vi "Dashboard Main.vi"() -> ()   [LabVIEW 2020]
uses:
  <vilib>/event_ctls.llb/eventvkey.ctl
  <vilib>/Rock Robotics/Network Tables/NT Read Numeric Array.vi
  <vilib>/Rock Robotics/WPI/Dashboard/WPI_DashboardLogging Global.vi
panel:
  out "Camera Perf":string
  in  "Camera Settings":T1={"Frame Rate"=30, "Compression"=30, "Size"=1, "DB Camera Config"=FALSE} {"Frame Rate" scale=1.0..30.0; "Compression" scale=100.0..-1.0; "Size" items=["640x480", "320x240", "160x120"]}
  in  "TCP":refnum<k5>
  in  "Rec Mode":enum32{"Stop", "Record", "Playback"}(radio)
  out "Robot IP":string
  out "Image Message":string="Timeout in Camera Communications"
  in  "Dashboard Tab":T2(tab)
  in  "Select Auto":string(combo)="Select Autonomous ..."
  out "NT Connection":bool
  out "MotorChart R":cluster{"Numeric":dbl, "Numeric":dbl}(graph)
  out "MotorChart L":cluster{"Numeric":dbl, "Numeric":dbl}(graph)
  out "MotorSliders R":cluster{"MotorSlide1":dbl, "MotorSlide2":dbl} {"MotorSlide2" scale=-1.0..1.0 scale format="%#_2e"; "MotorSlide1" scale=-1.0..1.0 scale format="%#_2e"}
  out "MotorSliders L":cluster{"MotorSlide1":dbl, "MotorSlide2":dbl} {"MotorSlide2" scale=-1.0..1.0 scale format="%#_2e"; "MotorSlide1" scale=-1.0..1.0 scale format="%#_2e"}
  out "Gyro":dbl(knob) scale=0.0..360.0
  out "JS1 Z":dbl(slide) scale=-1.0..1.0 scale format="%#_2e"
  out "JS1 Graph":cluster{"X":dbl, "Y":dbl}[](graph)
  out "JS1 Buttons":T3
  out "JS2 Z":dbl(slide) scale=-1.0..1.0 scale format="%#_2e"
  out "JS2 Graph":cluster{"X":dbl, "Y":dbl}[](graph)
  out "JS2 Buttons":T3
  out "Mode":T4(ring)=enum."Auto Disabled"
  out "Right Camera Perf":cluster{"Bandwidth (Mbps)":dbl, "FPS":dbl}
  in  "DB/String 9":string
  in  "DB/String 8":string
  in  "DB/String 7":string
  in  "DB/String 6":string
  in  "DB/String 5":string
  in  "DB/String 4":string
  in  "DB/String 3":string
  in  "DB/String 2":string
  in  "DB/String 1":string
  in  "DB/String 0":string
  in  "DB/Slider 0":dbl(slide) scale=0.0..5.0
  in  "DB/Slider 1":dbl(slide) scale=0.0..5.0
  in  "DB/Slider 2":dbl(slide) scale=0.0..5.0
  in  "DB/Slider 3":dbl(slide) scale=0.0..5.0
  out "DB/LED 3":bool
  out "DB/LED 2":bool
  out "DB/LED 1":bool
  out "DB/LED 0":bool
  in  "DB/Button 3":bool
  in  "DB/Button 2":bool
  in  "DB/Button 1":bool
  in  "DB/Button 0":bool caption="New Name"
  in  "Test Slider":dbl(slide) scale=0.0..100.0 scale format="%#_3g"
  in  "On/Off":bool caption="Solenoid"
  in  "Test Name":u16(ring) items=["Select the test to run..."]
  in  "Test Tree":string(tree)
  in  "Motor":cluster{"Value":dbl, "Enable":bool} {"Value" scale=-1.0..1.0 scale format="%#_3g"}
  out "Progress":T5 {"Test Progress" scale=0.0..100.0}
  in  "Rev/Fwd":cluster{"Forward":bool, "Reverse":bool}
  in  "Test Ring":u16(ring) items=["Monochrome", "Color"]
  in  "CheckList":i32(listbox)
  out "Tree":string(tree)
  out "Camera Image":T6(plugin-control)
  out "Background":bool
  in  "Camera Name":string(combo)="No Camera Selection"
  # "HW"
  # "Joysticks"
  # "Drive Motors"
  # "Front"
  # "Right"
  # "Left"
  # "Back"
  # "This tab is a great place for autonomous settings and robot-specific values.\nPlace controls and indicators inside this tab and match name to\nDashboard Variables on robot. You can also delete this comment."
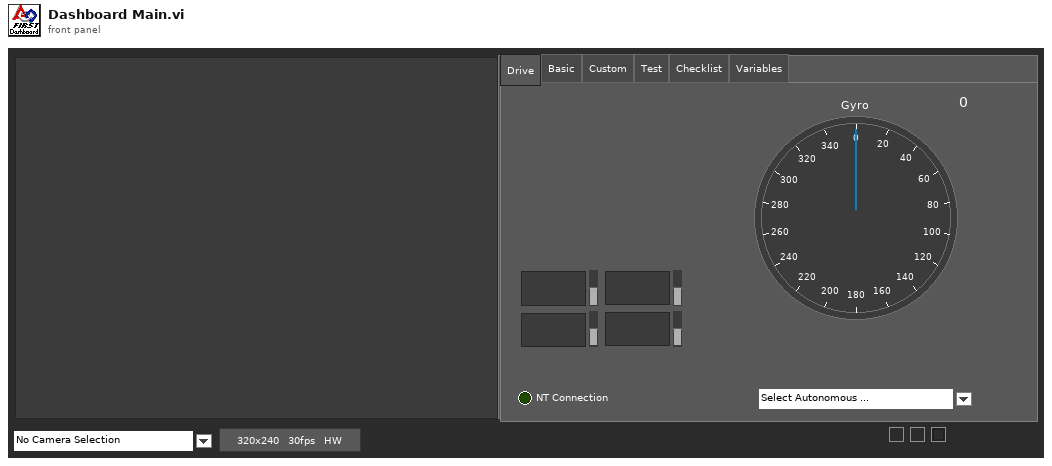
[diagram p1: front panel]
types:
  T1 = cluster{"Frame Rate":i32, "Compression":i32, "Size":u16, "DB Camera Config":bool}
  T2 = enum32{"Drive", "Basic", "Custom", "Test", "Checklist", "Variables"}
  T3 = cluster{bool, bool, bool, bool, bool, bool, bool, bool, bool, bool, bool, bool}
  T4 = enum8{"Tele-Op Disabled", "Tele-Op Enabled", "Auto Disabled", "Auto Enabled", "Test Disabled", "Test Enabled", "Disconnected", "No Code", "E-Stop"}
  T5 = cluster{"Test Progress":u8, "Test Progress Text":string}
  T6 = typedef "IMAQ Image.ctl" = refnum<image>
  T7 = cluster{"Save Path":path, "Interval (s)":dbl, "Keep":i32}
  T8 = enum32{"Drive", "Camera", "Basic", "Custom", "Test", "Commands", "Checklist", "Variables"}
  T9 = typedef "Image Type" = u32
  T10 = cluster{"Error Strings":string, "Disable Counts":cluster{u16, u16}, "Rail Faults":cluster{u16, u16, u16}, "Robot IP":string, "DB Mode":u8, "Event Info":cluster{"Name":string, "Type":u8, "Number":u16, "Replay":u8}}
  T11 = cluster{"Storage":cluster{"Disk Free":u64, "RAM Block":u32, "RAM free":u32}, "CPU Utilization":cluster{"CPU % ISR":sgl, "CPU % Time Crit":sgl, "CPU % Timed Str":sgl, "CPU % High":sgl, "CPU % Above":sgl, "CPU % Normal":sgl, "CPU % Low":sgl}, "CAN":cluster{"% Bus Utilization":sgl, "Bus Off Cnt":u32, "TX_FIFO Full Cnt":u32, "Receive Error Cnt":u8, "Transmit Error Cnt":u8}, "HID":cluster{"HID Outputs":u32, "Rumble Low":u16, "Rumble High":u16}[]}
  T12 = cluster{"Status bits":cluster{"Test Mode":bool, "Autonomous":bool, "Enabled":bool, "Code Start":bool, "Brownout":bool, "Reserved 2":bool, "Reserved 3":bool, "E-Stop":bool}, "Code Trace":cluster{"Disabled":bool, "TeleOp":bool, "Auto":bool, "Test":bool}, "Controller Type":enum16{"unknown", "cRIO", "roboRio"}, "Code?":enum16{"unknown", "noCode", "code"}, "Battery V":dbl}
  T13 = cluster{"Control Bits":cluster{"TestMode":bool, "Autonomous":bool, "Enabled":bool, "FMS Present":bool, bool, bool, bool, "E-Stop":bool}, "Team Station ":u8, "Countdown":sgl, "Joystick Values":cluster{"Axes":dbl[], "Buttons":bool[], "POVs":i16[]}[]}
  T14 = cluster{"Axes":dbl[], "Buttons":bool[], "POVs":i16[]}[]
  T15 = cluster{"Axes":dbl[], "Buttons":bool[], "POVs":i16[]}
  T16 = cluster{"Buttons[0]":bool, "Buttons[1]":bool, "Buttons[2]":bool, "Buttons[3]":bool, "Buttons[4]":bool, "Buttons[5]":bool, "Buttons[6]":bool, "Buttons[7]":bool, "Buttons[8]":bool, "Buttons[9]":bool, "Buttons[10]":bool, "Buttons[11]":bool}
  T17 = cluster{"Camera Image":refnum<vi>, "Dashboard Tab":refnum<vi>, "Background":refnum<vi>, "Rec Mode":refnum<vi>, "Test Slider":refnum<vi>, "On/Off ":refnum<vi>, "Test Ring":refnum<vi>, "Rev/Fwd":refnum<vi>, "Test Name":refnum<vi>, "Motor":refnum<vi>, "Progress":refnum<vi>, "CheckList":refnum<vi>, "Tree":refnum<vi>, "Test Tree":refnum<vi>, "Camera Settings":refnum<vi>, "Camera Name":refnum<vi>, "Camera Perf":refnum<vi>, "Camera Settings":refnum<vi>, "Camera Name":refnum<vi>, "Camera Image":refnum<vi>}
  T18 = cluster{"Global Rectangle":i32[], "Contours":cluster{"Contour Type":u32, "ROI Type":u32, "Points":i32[]}[]}
  T19 = cluster{"Camera Name":string, string, "Saved DB Images Info":cluster{"Save Path":path, "Interval (s)":dbl, "Keep":i32}}
  T20 = cluster{"Operation":enum16{"Update", "Clear"}, "Color Box":u32}[]
  T21 = typedef "eventvkey.ctl" = enum16{"ASCII", "Enter", "Return", "Shift", "Ctrl", "Alt", "Cmd", "Opt", "Caps", "NumLock", "Clear", "Break", "Up", "Down", "Left", "Right", "Insert", "Delete", "Home", "End", "PageUp", "PageDown", "Escape", "Help", "Pause", "ScrollLock", "F1", "F2", "F3", "F4", "F5", "F6", "F7", "F8", "F9", "F10", "F11", "F12", "F13", "F14", "F15", "F16", "F17", "F18", "F19", "F20", "F21", "F22", "F23", "F24", "Play", "VolumeUp", "VolumeDown", "Mute", "Two Byte Char"}
  T22 = cluster{"Image Size":bool, "Image Type":bool, "Pixel Value":bool, "ROI Information":bool, "Zoom Factor":bool}
  T23 = cluster{"Operation":enum16{"Update", "Clear"}, "Color Box":u32}
  T24 = cluster{"Shift":bool, "Ctrl":bool, "Alt":bool, "Cmd":bool, "Opt":bool}
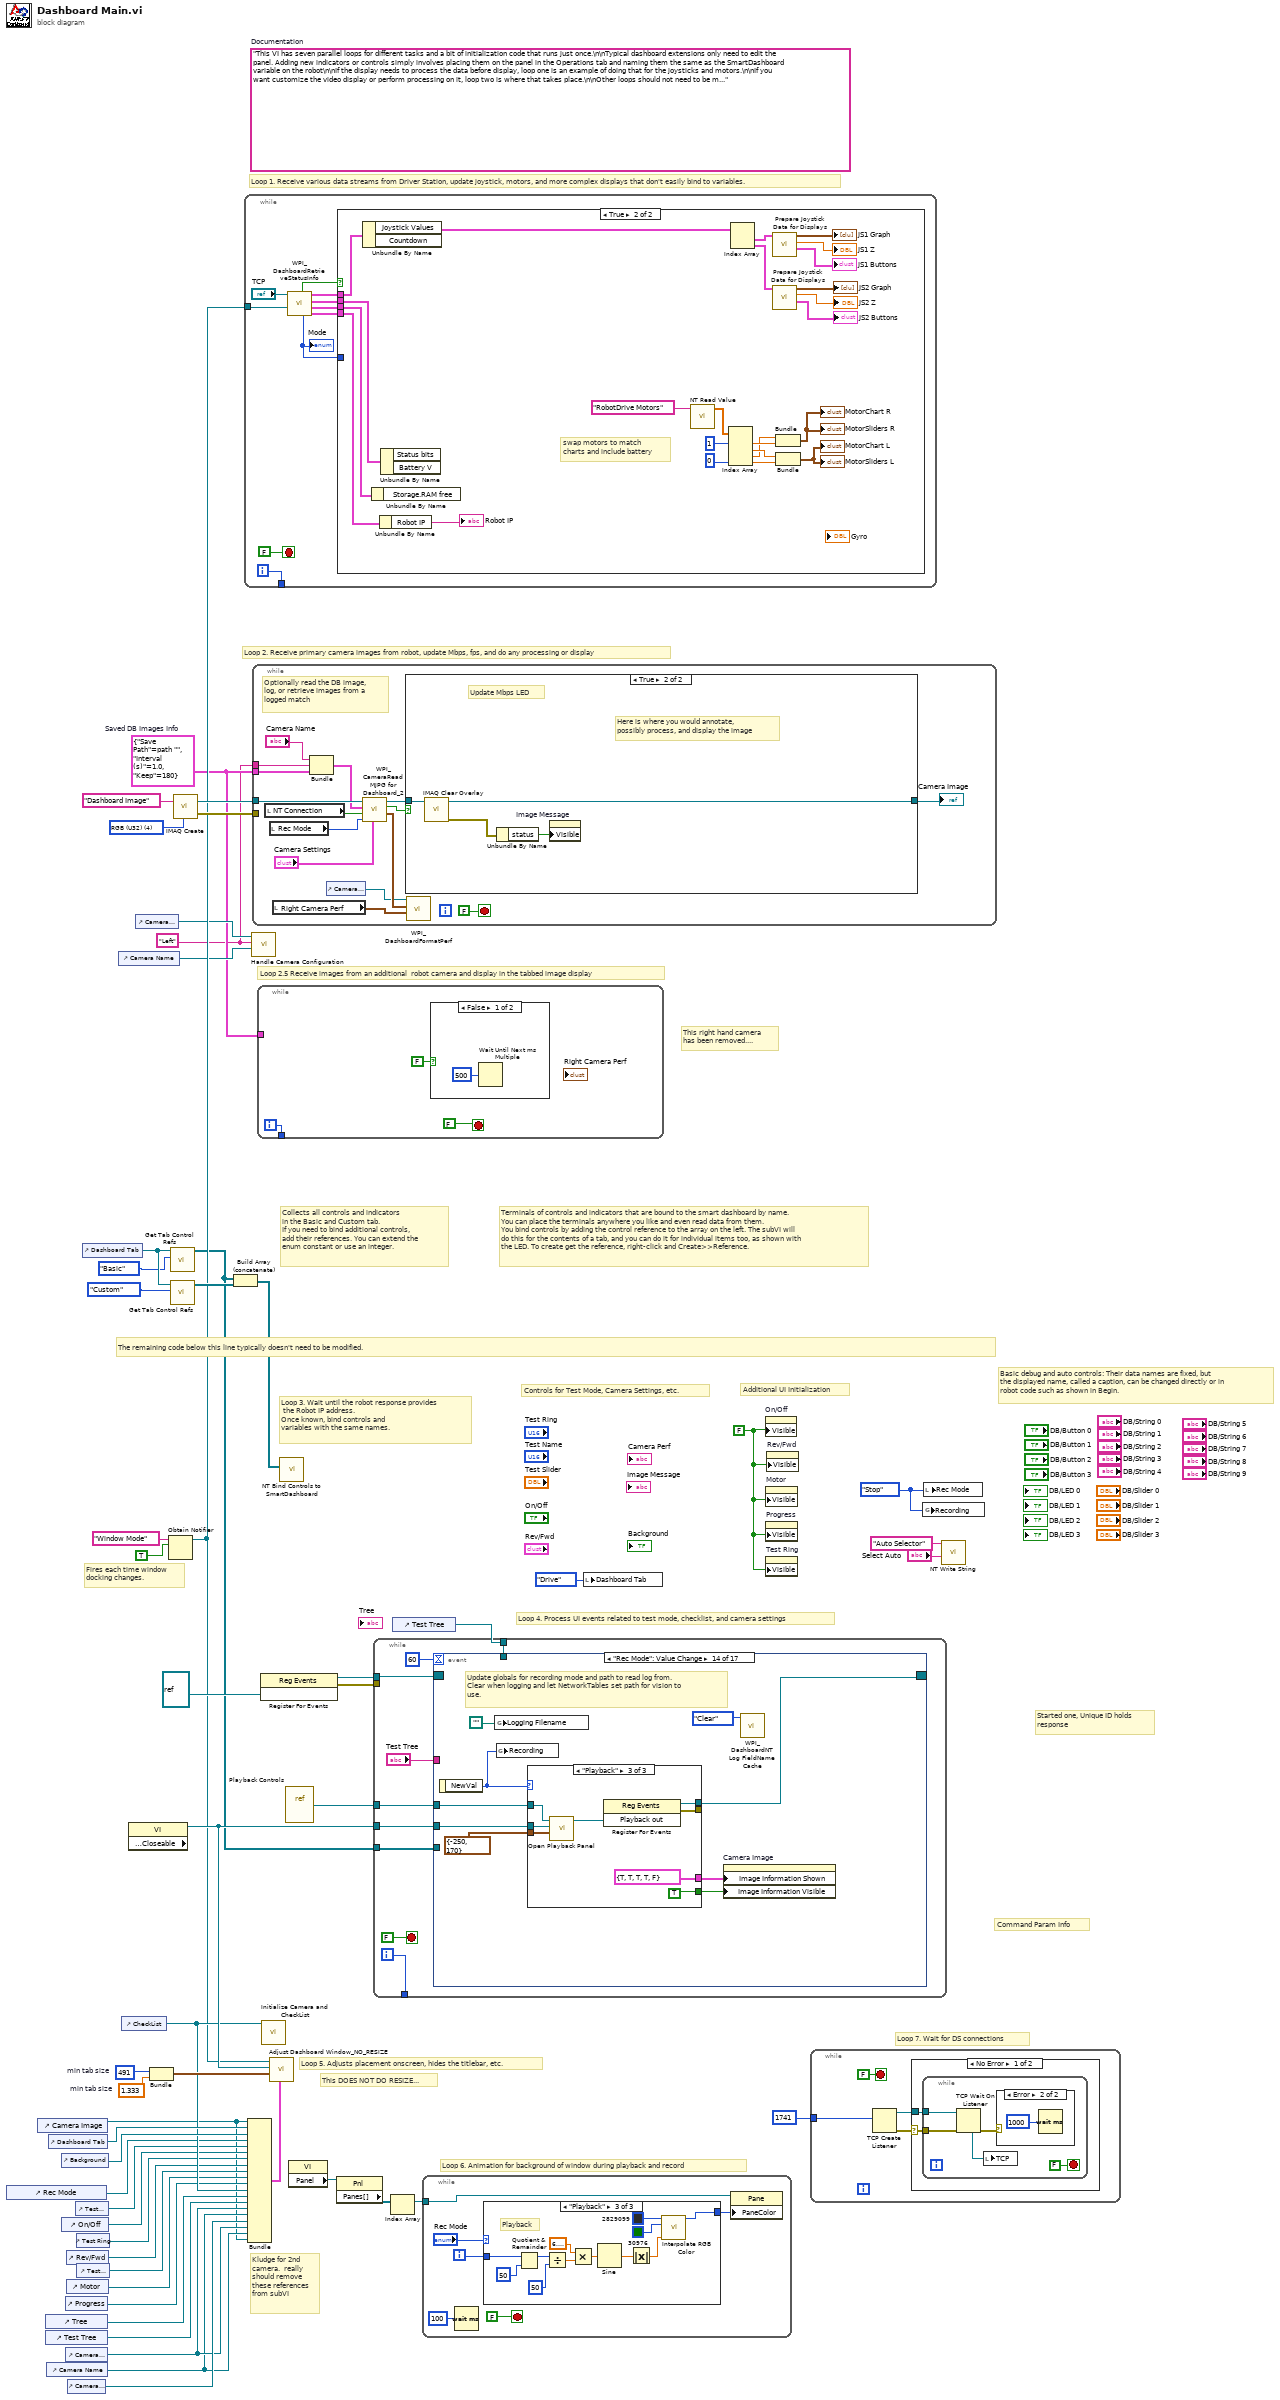
[diagram p0: block diagram]
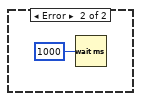
[diagram p4: hidden frame]
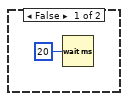
[diagram p5: hidden frame]
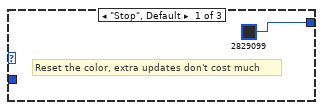
[diagram p6: hidden frame]
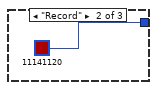
[diagram p7: hidden frame]
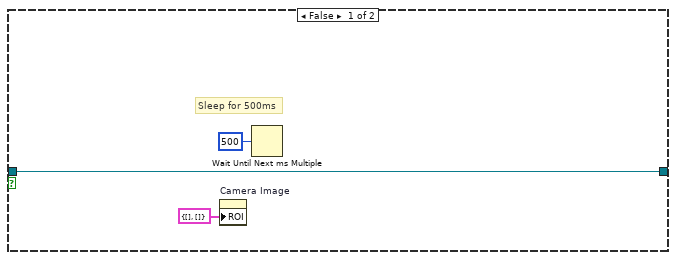
[diagram p8: hidden frame]
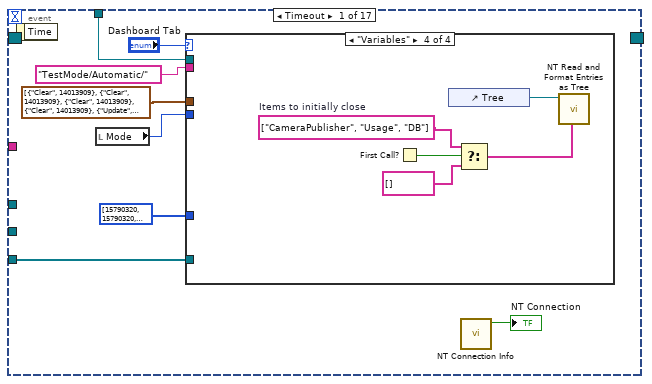
[diagram p9: hidden frame]
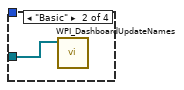
[diagram p11: hidden frame]
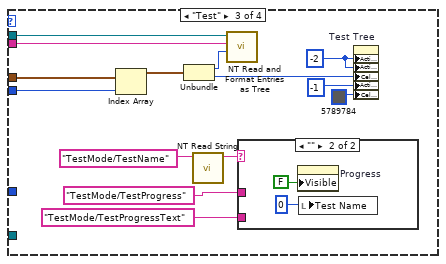
[diagram p12: hidden frame]
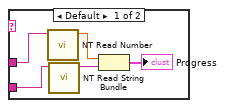
[diagram p13: hidden frame]
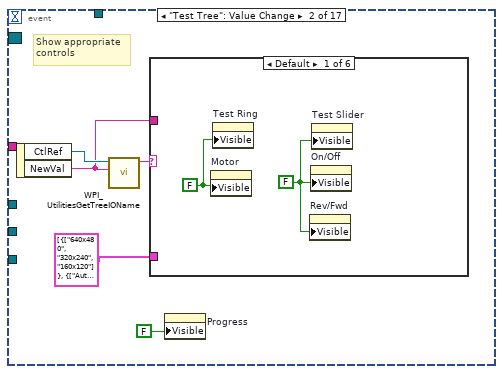
[diagram p14: hidden frame]
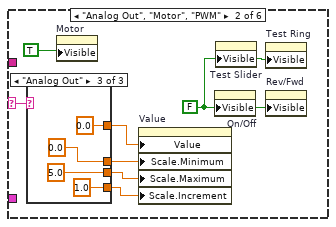
[diagram p15: hidden frame]
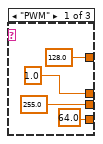
[diagram p16: hidden frame]
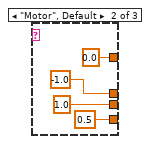
[diagram p17: hidden frame]
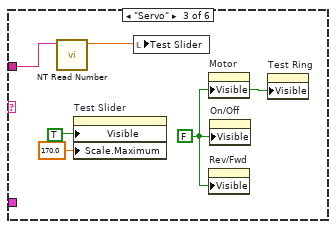
[diagram p18: hidden frame]
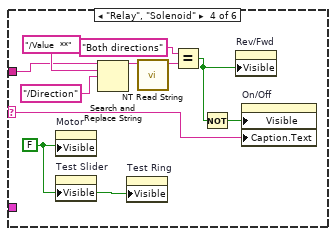
[diagram p19: hidden frame]
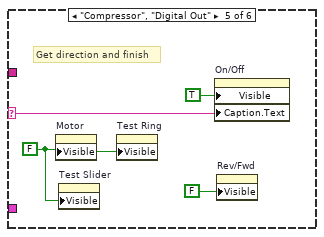
[diagram p20: hidden frame]
diagram:
  w6 = T7 {"Save Path"=path "", "Interval (s)"=1.0, "Keep"=180}  # Saved DB Images Info
  w5 = "Left"
  w33 = 491  # min tab size
  w32 = 1.333  # min tab size
  w39 = enum32{"Stop", "Record", "Playback"}."Stop" ("Rec Mode")
  w17 = FALSE ("Visible")
  (unwired) "This VI has seven parallel loops for different tasks and a bit of initialization code that runs just once.\n\nTypical dashboard extensions only need to edit the panel. Adding new indicators or controls simply involves placing them on the panel in the Operations tab and naming them the same as the SmartDashboard variable on the robot\n\nIf the display needs to process the data before display, loop one is an example of doing that for the joysticks and motors.\n\nIf you want customize the video display or perform processing on it, loop two is where that takes place.\n\nOther loops should not need to be modified. They are pretty standard, and document the task they perform."  # Documentation
  w53 = T9 4 items=["Grayscale (U8)", "Grayscale (I16)", "Grayscale (SGL)", "Complex (CSG)", "RGB (U32)", "HSL (U32)", "RGB (U64)"] ("Image Type")
  # "Kludge for 2nd\ncamera.  really\nshould remove\nthese references\nfrom subVI"
  # "This right hand camera\nhas been removed...."
  # "This DOES NOT DO RESIZE..."
  # "Loop 2.5 Receive images from an additional  robot camera and display in the tabbed image display"
  # "Command Param Info"
  # "Started one, Unique ID holds\nresponse"
  # "Loop 7. Wait for DS connections"
  # "Basic debug and auto controls: Their data names are fixed, but\nthe displayed name, called a caption, can be changed directly or in\nrobot code such as shown in Begin."
  # "Controls for Test Mode, Camera Settings, etc."
  # "Additional UI Initialization"
  # "Loop 6. Animation for background of window during playback and record"
  # "Fires each time window\ndocking changes."
  # "Collects all controls and indicators\nin the Basic and Custom tab.\nIf you need to bind additional controls,\nadd their references. You can extend the\nenum constant or use an integer."
  # "The remaining code below this line typically doesn't need to be modified."
  # "Loop 4. Process UI events related to test mode, checklist, and camera settings"
  # "Terminals of controls and indicators that are bound to the smart dashboard by name.\nYou can place the terminals anywhere you like and even read data from them.\nYou bind controls by adding the control reference to the array on the left. The subVI will\ndo this for the contents of a tab, and you can do it for individual items too, as shown with\nthe LED. To create get the reference, right-click and Create>>Reference."
  # "Loop 3. Wait until the robot response provides\n the Robot IP address.\nOnce known, bind controls and\nvariables with the same names."
  # "Loop 5. Adjusts placement onscreen, hides the titlebar, etc."
  # "Loop 1. Receive various data streams from Driver Station, update joystick, motors, and more complex displays that don't easily bind to variables."
  # "Loop 2. Receive primary camera images from robot, update Mbps, fps, and do any processing or display"
  n1 = control-ref of="Rec Mode"() -> (w23:refnum<vi>)
  n2 = control-ref of="Camera Image"() -> (w2:refnum<vi>)
  n3 = control-ref of="Tree"() -> (w27:refnum<vi>)
  n4 = control-ref of="Test Tree"() -> (w26:refnum<vi>)
  n5 = control-ref of="Camera Name"() -> (w3:refnum<vi>)
  n6 = control-ref of="Dashboard Tab"() -> (w34:refnum<vi>)
  n7 = control-ref of="Background"() -> (w30:refnum<vi>)
  n8 = control-ref of="On/Off"() -> (w21:refnum<vi>)
  n9 = control-ref of="Progress"() -> (w18:refnum<vi>)
  n10 = control-ref of="Camera Settings"() -> (w4:refnum<vi>)
  n11 = control-ref of="Rev/Fwd"() -> (w19:refnum<vi>)
  n12 = control-ref of="Motor"() -> (w24:refnum<vi>)
  n13 = control-ref of="Camera Perf"() -> (w12:refnum<vi>)
  n14 = control-ref of="Test Slider"() -> (w22:refnum<vi>)
  n15 = control-ref of="Test Ring"() -> (w20:refnum<vi>)
  n16 = control-ref of="Test Name"() -> (w25:refnum<vi>)
  n17 = control-ref of="Dashboard Tab"() -> (w37:refnum<vi>)
  n18 = control-ref of="Camera Name"() -> (w13:refnum<vi>)
  n19 = control-ref of="CheckList"() -> (w28:refnum<vi>)
  n20 = property class="VI" props=["Front Panel.Closeable"]() -> (reference out=w38:refnum<vi>)  [unwired: 2 in, 2 out]
  n21 = control-ref of="Camera Settings"() -> (w14:refnum<vi>)
  n22 = Bundle("min tab size"=w33, "min tab size"=w32) -> (w31:cluster{"min tab size":i32, "min tab size":dbl})  [unwired: 1 in]
  n23 = Obtain Notifier(name (unnamed)="Window Mode", notification data type=TRUE) -> (notifier out=w16:refnum<notifier>)  [unwired: 2 in, 2 out]
  n24 = call <vilib>:"Get Tab Control Refs.vi"("Page Index"=T8."Basic" ("Dashboard Tab"), "TabControl in"=w37) -> ("ControlsOnPage"=w11:refnum<vi>[])  [unwired: 9 in]
  n25 = call <vilib>:"Get Tab Control Refs.vi"("Page Index"=T8."Custom" ("Dashboard Tab"), "TabControl in"=w37) -> ("ControlsOnPage"=w36:refnum<vi>[])  [unwired: 9 in]
  n26 = call "IMAQ Create"("Image Name"="Dashboard Image", "Image Type"=w53) -> ("New Image"=w51:T6, "error out"=w50:errorcluster)  [unwired: 2 in, 1 out]
  n27 = Build Array (concatenate)(w11, w36) -> (w35:refnum<vi>[])
  n28 = while {
    tunnel: [w62] -> _
    tunnel: w16 -> [w54]
    i -> [w62]
    stop <- FALSE stop-if-true
    n29 = call <vilib>:"WPI_DashboardRetrieveStatusInfo.vi"("Window Mode Notifier"=w54, "TCP Cnx"="TCP") -> ("Power and Errors"=w57:T10, "Robot Metrics"=w60:T11, "Status Info"=w61:T12, "Control Info"=w58:T13, "Robot Mode"=w56:T4, "Process?"=w59:bool)  [unwired: 4 in]
    "Mode" <- w56
    n30 = case shown="True" w59 {
      tunnel: w61 -> [_ w88]
      tunnel: w60 -> [_ w87]
      tunnel: w58 -> [_ w86]
      tunnel: w57 -> [_ w85]
      tunnel: w56 -> [_ _]
      frame False {
        n31 = Wait (ms)(milliseconds to wait=u32 20) -> ()  [unwired: 1 out]
      }
      frame True {
        # "swap motors to match\ncharts and include battery"
        n32 = Unbundle By Name(w86) -> ("Joystick Values"=w76:T14)  [unwired: 1 out]
        n33 = Unbundle By Name(w87) -> ()  [unwired: 1 out]
        n34 = Unbundle By Name(w85) -> ("Robot IP"=→"Robot IP":string)
        n35 = Unbundle By Name(w88) -> ()  [unwired: 2 out]
        n36 = call-poly <vilib>:"NT Read Value.vi"("name"="RobotDrive Motors" ("Name")) -> ("value"=w66:dbl[])  [unwired: 8 in, 2 out]
        n37 = Index Array(array=w66, index #1=1, index #4=0) -> (element #1=w80:dbl, element #2=w81:dbl, element #3=w79:dbl, element #4=w84:dbl)  [unwired: 2 in]
        n38 = Index Array(array=w76) -> (element #1=w75:T15, element #2=w71:T15)  [unwired: 2 in]
        n39 = call "Prepare Joystick Data for Displays.vi"("Joystick Values"=w71) -> ("Buttons"=→"JS2 Buttons":T16, "Z Axis"=→"JS2 Z":dbl, "Cartesian Data"=→"JS2 Graph":cluster{"X axis":dbl, "X axis":dbl}[])  [unwired: 8 in]
        n40 = call "Prepare Joystick Data for Displays.vi"("Joystick Values"=w75) -> ("Buttons"=→"JS1 Buttons":T16, "Z Axis"=→"JS1 Z":dbl, "Cartesian Data"=→"JS1 Graph":cluster{"X axis":dbl, "X axis":dbl}[])  [unwired: 8 in]
        n41 = Bundle("Numeric"=w79, "Numeric"=w80) -> (→"MotorChart R" →"MotorSliders R":cluster{"Numeric":dbl, "Numeric":dbl})  [unwired: 1 in]
        n42 = Bundle("Numeric"=w81, "Numeric"=w84) -> (→"MotorChart L" →"MotorSliders L":cluster{"Numeric":dbl, "Numeric":dbl})  [unwired: 1 in]
      }
    }
  }
  n43 = Bundle("Camera Image"=w2, "Dashboard Tab"=w34, "Background"=w30, "Rec Mode"=w23, "Test Slider"=w22, "On/Off"=w21, "Test Ring"=w20, "Rev/Fwd"=w19, "Test Name"=w25, "Motor"=w24, "Progress"=w18, "CheckList"=w28, "Tree"=w27, "Test Tree"=w26, "Camera Settings"=w4, "Camera Name"=w3, "Camera Perf"=w12, "Camera Settings"=w4, "Camera Name"=w3, "Camera Image"=w2) -> (w29:T17)  [unwired: 1 in]
  n44 = call "Handle Camera Configuration.vi"("CameraNameRef"=w13, "Display Name"=w5, "ClusterRef"=w14) -> ()  [unwired: 9 in]
  n45 = while {
    tunnel: w51 -> [w102]
    tunnel: w50 -> [_]
    tunnel: w6 -> [w95]
    tunnel: w5 -> [w92]
    stop <- FALSE stop-if-true
    # "Optionally read the DB image,\nlog, or retrieve images from a\nlogged match"
    n46 = local read "NT Connection"() -> (w96:bool)
    n47 = local read "Rec Mode"() -> (w99:enum32{"Stop", "Record", "Playback"})
    n48 = local read "Right Camera Perf"() -> (w90:cluster{"Bandwidth (Mbps)":dbl, "FPS":dbl})
    n49 = Bundle("Camera Name"="Camera Name", w92, "Saved DB Images Info"=w95) -> (w94:T19)  [unwired: 1 in]
    n50 = control-ref of="Camera Perf"() -> (w89:refnum<vi>)
    n51 = call <vilib>:"WPI_CameraRead MJPG for Dashboard_2.vi"("Camera Settings"="Camera Settings", "Rec Mode"=w99, "NT Connection"=w96, "Capture Info"=w94, "Image in"=w102) -> ("perf info"=w91:cluster{"Bandwidth (Mbps)":dbl, "fps":dbl}, "Active"=w100:bool, "Image\\ out"=w101:T6)  [unwired: 4 in]
    n52 = case shown="True" w100 {
      tunnel: w101 -> [w105 w108]
      tunnel: [w105 w107] -> w97
      frame False {
        # "Sleep for 500ms"
        n53 = property on="Camera Image" class="ImageControl"("ROI"=T18 {"Global Rectangle"=[], "Contours"=[]}) -> ()  [unwired: 2 in, 2 out]
        n54 = Wait Until Next ms Multiple(millisecond multiple=u32 500) -> ()  [unwired: 1 out]
      }
      frame True {
        # "Here is where you would annotate,\npossibly process, and display the image"
        # "Update Mbps LED"
        n55 = call "IMAQ Clear Overlay"("Image"=w108) -> ("error out"=w109:errorcluster, "Image Out"=w107:T6)  [unwired: 2 in, 7 out]
        n56 = Unbundle By Name(w109) -> ("status"=w110:bool)
        n57 = property on="Image Message" class="Str"("Visible"=w110) -> ()  [unwired: 2 in, 2 out]
      }
    }
    "Camera Image" <- w97
    n58 = call <vilib>:"WPI_DashboardFormatPerf.vi"("Right Camera Perf"=w90, "Performance"=w91, "String in"=w89) -> ()  [unwired: 9 in]
  }
  n59 = while {
    tunnel: [w112] -> _
    tunnel: w6 -> [_]
    i -> [w112]
    stop <- FALSE stop-if-true
    n60 = case shown="False" FALSE {
      frame False {
        n61 = Wait Until Next ms Multiple(millisecond multiple=u32 500) -> ()  [unwired: 1 out]
      }
      frame True {
      }
    }
  }
  n62 = register-events(refnum<vi> refnum) -> (reference out=w42:refnum<event-registration>, error out=w41:errorcluster)  [unwired: 2 in]
  n63 = call "Initialize Camera and CheckList.vi"("ListBox in"=w28) -> ()  [unwired: 11 in]
  n64 = call "Adjust Dashboard Window_NO_RESIZE.vi"("Sizing Refnums"=w29, "Size Constraints"=w31, "VI"=w38, "WIn Mode"=w16) -> ()  [unwired: 8 in]
  n65 = call <vilib>:"NT Bind Controls to SmartDashboard.vi"("Bound Control Refs"=w35) -> ()  [unwired: 11 in]
  n66 = vi-ref "Playback Controls.vi"() -> (w43:refnum<vi>)
  n67 = property class="VI"() -> ("Panel"=w45:refnum<vi>)  [unwired: 2 in, 2 out]
  n68 = property class="Pnl"(reference=w45) -> ("Panes[]"=w46:refnum<vi>[])  [unwired: 1 in, 2 out]
  n69 = Index Array(array=w46) -> (element=w44:refnum<vi>)  [unwired: 1 in]
  n70 = control-ref of="Test Tree"() -> (w47:refnum<vi>)
  n71 = while {
    tunnel: [w120] -> _
    tunnel: w47 -> [w119]
    tunnel: w43 -> [w118]
    tunnel: w42 -> [w117]
    tunnel: w41 -> [_]
    tunnel: w38 -> [w116]
    tunnel: w11 -> [w115]
    i -> [w120]
    stop <- FALSE stop-if-true
    n72 = event shown="[13] \"Rec Mode\": Value Change" {
      selector: w117 -> [_ _ _ _ _ _ _ _ _ _ _ _ _ _ _ _ _]
      dyn-events: [_ _ _ _ _ _ _ _ _ _ _ _ _ w325 _ _ _] -> _
      timeout: u32 60 ("milliseconds to wait") -> [_ _ _ _ _ _ _ _ _ _ _ _ _ _ _ _ _]
      tunnel: w119 -> [w130 _ _ _ _ _ _ _ _ _ _ _ _ _ _ _ _]
      tunnel: "Test Tree" -> [_ _ _ _ _ _ _ _ w298 w305 w306 w309 w316 _ _ _ _]
      tunnel: w118 -> [_ _ _ _ _ _ _ _ _ _ _ _ _ w327 _ w342 _]
      tunnel: w116 -> [_ _ _ _ _ _ _ _ _ _ _ _ _ w323 _ _ _]
      tunnel: w115 -> [w125 _ _ _ _ _ _ _ _ _ _ _ _ _ _ _ _]
      event Timeout {
        n73 = event-data() -> ()  [unwired: 1 in, 1 out]
        n74 = local read "Mode"() -> (w128:T4)
        n75 = case shown="\"Variables\"" "Dashboard Tab" {
          tunnel: w130 -> [_ _ w146 _]
          tunnel: "TestMode/Automatic/" ("Name Pattern") -> [_ _ w145 _]
          tunnel: T20 [{"Operation"=enum."Clear", "Color Box"=14013909}, {"Operation"=enum."Clear", "Color Box"=14013909}, {"Operation"=enum."Clear", "Color Box"=14013909}, {"Operation"=enum."Clear", "Color Box"=14013909}, {"Operation"=enum."Update", "Color Box"=14013909}, {"Operation"=enum."Update", "Color Box"=16777215}, {"Operation"=enum."Clear", "Color Box"=14013909}, {"Operation"=enum."Clear", "Color Box"=14013909}, {"Operation"=enum."Clear", "Color Box"=14013909}] -> [_ _ w138 _]
          tunnel: w128 -> [_ _ w137 _]
          tunnel: u32[] [15790320, 15790320, 15790320, 15790320, 16777215, 16777215, 15790320, 15790320, 15790320] -> [_ _ _ _]
          tunnel: w125 -> [_ w132 _ _]
          frame "Custom", Default {
          }
          frame "Basic" {
            n76 = call <vilib>:"WPI_DashboardUpdateNames.vi"("Controls on Tab"=w132) -> ()  [unwired: 11 in]
          }
          frame "Test" {
            w144 = -2 ("Active Item:Row Number")
            n77 = Index Array(array=w138, index=w137) -> (element=w139:T23)
            n78 = Unbundle(w139) -> ("Operation"=w140:enum16{"Update", "Clear"}, "Color Box"=w141:u32)
            n79 = call <vilib>:"NT Read String.vi"("name"="TestMode/TestName" ("Name")) -> ("value"=w135:string)  [unwired: 8 in, 2 out]
            n80 = call <vilib>:"NT Read and Format Entries as Tree.vi"("Operation"=w140, "Name Pattern"=w145, "Tree Refnum"=w146) -> ()  [unwired: 7 in, 2 out]
            n81 = case shown="\"\"" w135 {
              tunnel: "TestMode/TestProgress" ("Name") -> [w148 _]
              tunnel: "TestMode/TestProgressText" ("Name") -> [w147 _]
              frame Default {
                n82 = call <vilib>:"NT Read Number.vi"("name"=w148) -> ("value"=w149:dbl)  [unwired: 8 in, 2 out]
                n83 = call <vilib>:"NT Read String.vi"("name"=w147) -> ("value"=w150:string)  [unwired: 8 in, 2 out]
                n84 = Bundle("value"=w149, "value"=w150) -> (→"Progress":cluster{"value":dbl, "value":string})  [unwired: 1 in]
              }
              frame "" {
                n85 = property on="Progress" class="Clust (strict)"("Visible"=FALSE) -> ()  [unwired: 2 in, 2 out]
                n86 = local write "Test Name"(u16 0) -> ()
              }
            }
            n87 = property on="Test Tree" class="Tree (strict)"("Active Item Row Number"=w144, "ActiveColNum"=w144, "CellBG"=w141, "Active Item Row Number"=-1 ("Active Item:Row Number"), "CellBG"=u32 5789784 ("Color Box")) -> ()  [unwired: 2 in, 2 out]
          }
          frame "Variables" {
            w156 = string[] ["CameraPublisher", "Usage", "DB"]  # Items to initially close
            n88 = First Call?() -> (First Call?: T/F=w157:bool)
            n89 = control-ref of="Tree"() -> (w158:refnum<vi>)
            n90 = Select(t=w156, s=w157, f=string[] []) -> (s? t:f=w154:string[])
            n91 = call <vilib>:"NT Read and Format Entries as Tree.vi"("Tags to  Close"=w154, "Tree Refnum"=w158) -> ()  [unwired: 8 in, 2 out]
          }
        }
        n92 = call <vilib>:"NT Connection Info.vi"() -> ("Connected"=→"NT Connection":bool)  [unwired: 11 in]
      }
      event "Test Tree": Value Change {
        # "Show appropriate\ncontrols"
        n93 = event-data() -> ("CtlRef"=w162:refnum<vi>, "NewVal"=w160:string)  [unwired: 1 in]
        n94 = call <vilib>:"WPI_UtilitiesGetTreeIOName.vi"("NewVal"=w160, "TreeControl in"=w162) -> ("I/O Name"=w163:string)  [unwired: 9 in]
        n95 = case shown="Default" w163 {
          selector: w163 -> [_ w170 _ w192 w201 _]
          tunnel: w160 -> [_ _ w189 w191 _ w208]
          tunnel: cluster{string[]}[] [{["640x480", "320x240", "160x120"]}, {["Auto", "Fixed indoor", "Fixed outdoor 1", "Fixed outdoor 2", "Fixed fluorescent 1", "Fixed fluorescent 2", "Hold current"]}, {["Auto", "Flicker-free 50 Hz", "Flicker-free 60 Hz", "Hold current"]}, {["None", "Prioritize frame rate", "Prioritize image quality"]}, {["Monochrome", "Color"]}] -> [_ _ _ _ _ w207]
          frame Default {
            w165 = FALSE ("Visible")
            w164 = FALSE ("Visible")
            n96 = property on="Motor" class="Clust (strict)"("Visible"=w164) -> ()  [unwired: 2 in, 2 out]
            n97 = property on="Test Ring" class="Ring (strict)"("Visible"=w164) -> ()  [unwired: 2 in, 2 out]
            n98 = property on="Rev/Fwd" class="Clust (strict)"("Visible"=w165) -> ()  [unwired: 2 in, 2 out]
            n99 = property on="On/Off" class="Bool (strict)"("Visible"=w165) -> ()  [unwired: 2 in, 2 out]
            n100 = property on="Test Slider" class="Slide (strict)"("Visible"=w165) -> ()  [unwired: 2 in, 2 out]
          }
          frame "Analog Out", "Motor", "PWM" {
            w171 = FALSE ("Visible")
            n101 = case shown="\"Analog Out\"" w170 {
              tunnel: [1.0 ("Value") -1.0 ("Value") 0.0 ("Value")] -> w169
              tunnel: [255.0 ("Value") 1.0 ("Value") 5.0 ("Value")] -> w168
              tunnel: [128.0 ("Value") 0.0 ("Value") 0.0 ("Value")] -> w167
              tunnel: [64.0 ("Value") 0.5 ("Value") 1.0 ("Value")] -> w166
              frame "PWM" {
              }
              frame "Motor", Default {
              }
              frame "Analog Out" {
              }
            }
            n102 = property on="Motor" class="Clust (strict)"("Visible"=TRUE) -> ()  [unwired: 2 in, 2 out]
            n103 = property on="Value" class="Slide (strict)"("Value"=w167, "Scale.Minimum"=w169, "Scale.Maximum"=w168, "Scale.Increment"=w166) -> ()  [unwired: 2 in, 2 out]
            n104 = property on="On/Off" class="Bool (strict)"("Visible"=w171) -> ()  [unwired: 2 in, 2 out]
            n105 = property on="Test Slider" class="Slide (strict)"("Visible"=w171) -> ()  [unwired: 2 in, 2 out]
            n106 = property on="Test Ring" class="Ring (strict)"("Visible"=w171) -> ()  [unwired: 2 in, 2 out]
            n107 = property on="Rev/Fwd" class="Clust (strict)"("Visible"=w171) -> ()  [unwired: 2 in, 2 out]
          }
          frame "Servo" {
            w187 = FALSE ("Visible")
            n108 = call <vilib>:"NT Read Number.vi"("name"=w189) -> ("value"=w188:dbl)  [unwired: 8 in, 2 out]
            n109 = property on="Test Slider" class="Slide (strict)"("Visible"=TRUE, "Scale.Maximum"=170.0 ("Scale.Range:Maximum")) -> ()  [unwired: 2 in, 2 out]
            n110 = local write "Test Slider"(w188) -> ()
            n111 = property on="Motor" class="Clust (strict)"("Visible"=w187) -> ()  [unwired: 2 in, 2 out]
            n112 = property on="Rev/Fwd" class="Clust (strict)"("Visible"=w187) -> ()  [unwired: 2 in, 2 out]
            n113 = property on="On/Off" class="Bool (strict)"("Visible"=w187) -> ()  [unwired: 2 in, 2 out]
            n114 = property on="Test Ring" class="Ring (strict)"("Visible"=w187) -> ()  [unwired: 2 in, 2 out]
          }
          frame "Relay", "Solenoid" {
            w190 = FALSE ("Visible")
            n115 = property on="Motor" class="Clust (strict)"("Visible"=w190) -> ()  [unwired: 2 in, 2 out]
            n116 = property on="Test Slider" class="Slide (strict)"("Visible"=w190) -> ()  [unwired: 2 in, 2 out]
            n117 = Search and Replace String(input string=w191, search string="/Value  **", replace string="/Direction") -> (result string=w197:string)  [unwired: 5 in, 3 out]
            n118 = property on="Test Ring" class="Ring (strict)"("Visible"=w190) -> ()  [unwired: 2 in, 2 out]
            n119 = call <vilib>:"NT Read String.vi"("name"=w197) -> ("value"=w195:string)  [unwired: 8 in, 2 out]
            n120 = Equal?(x="Both directions", y=w195) -> (x = y?=w193:bool)
            n121 = Not(x=w193) -> (.not. x?=w194:bool)
            n122 = property on="Rev/Fwd" class="Clust (strict)"("Visible"=w193) -> ()  [unwired: 2 in, 2 out]
            n123 = property on="On/Off" class="Bool (strict)"("Visible"=w194, "Caption.Text"=w192) -> ()  [unwired: 2 in, 2 out]
          }
          frame "Compressor", "Digital Out" {
            w200 = FALSE ("Visible")
            # "Get direction and finish"
            n124 = property on="Motor" class="Clust (strict)"("Visible"=w200) -> ()  [unwired: 2 in, 2 out]
            n125 = property on="Test Slider" class="Slide (strict)"("Visible"=w200) -> ()  [unwired: 2 in, 2 out]
            n126 = property on="Test Ring" class="Ring (strict)"("Visible"=w200) -> ()  [unwired: 2 in, 2 out]
            n127 = property on="On/Off" class="Bool (strict)"("Visible"=TRUE, "Caption.Text"=w201) -> ()  [unwired: 2 in, 2 out]
            n128 = property on="Rev/Fwd" class="Clust (strict)"("Visible"=FALSE) -> ()  [unwired: 2 in, 2 out]
          }
          frame "Camera" {
            n129 = call <vilib>:"NT_Get Last Path Segment.vi"("String in"=w208) -> ("String out"=w209:string)  [unwired: 10 in]
            n130 = property on="On/Off" class="Bool (strict)"("Visible"=FALSE) -> ()  [unwired: 2 in, 2 out]
            n131 = property on="Motor" class="Clust (strict)"("Visible"=FALSE) -> ()  [unwired: 2 in, 2 out]
            n132 = property on="Rev/Fwd" class="Clust (strict)"("Visible"=FALSE) -> ()  [unwired: 2 in, 2 out]
            n133 = case shown="\"White Balance  **\"" w209 {
              tunnel: w208 -> [w215 w224 w233 w242 w251 _ w257]
              tunnel: w207 -> [w213 w221 w230 w239 w248 _ _]
              frame "Size  **" {
                n134 = Index Array(array=w213) -> (element=w212:cluster{string[]})  [unwired: 1 in]
                n135 = call <vilib>:"NT Read String.vi"("name"=w215) -> ("value"=w214:string)  [unwired: 8 in, 2 out]
                n136 = Unbundle(w212) -> (w210:string[])
                n137 = Match First String(2:w210, 3:w214) -> (0:w211:i32)  [unwired: 1 out]
                n138 = property on="Test Ring" class="Ring (strict)"("Value"=w211, "Strings []"=w210) -> ()  [unwired: 2 in, 2 out]
                n139 = property on="Test Ring" class="Ring (strict)"("Visible"=TRUE) -> ()  [unwired: 2 in, 2 out]
                n140 = property on="Test Slider" class="Slide (strict)"("Visible"=FALSE) -> ()  [unwired: 2 in, 2 out]
              }
              frame "White Balance  **" {
                n141 = Index Array(array=w221, index=1) -> (element=w222:cluster{string[]})
                n142 = call <vilib>:"NT Read String.vi"("name"=w224) -> ("value"=w223:string)  [unwired: 8 in, 2 out]
                n143 = Unbundle(w222) -> (w219:string[])
                n144 = Match First String(2:w219, 3:w223) -> (0:w218:i32)  [unwired: 1 out]
                n145 = property on="Test Ring" class="Ring (strict)"("Value"=w218, "Strings []"=w219) -> ()  [unwired: 2 in, 2 out]
                n146 = property on="Test Ring" class="Ring (strict)"("Visible"=TRUE) -> ()  [unwired: 2 in, 2 out]
                n147 = property on="Test Slider" class="Slide (strict)"("Visible"=FALSE) -> ()  [unwired: 2 in, 2 out]
              }
              frame "Exposure  **" {
                n148 = Index Array(array=w230, index=2) -> (element=w231:cluster{string[]})
                n149 = call <vilib>:"NT Read String.vi"("name"=w233) -> ("value"=w232:string)  [unwired: 8 in, 2 out]
                n150 = Unbundle(w231) -> (w227:string[])
                n151 = Match First String(2:w227, 3:w232) -> (0:w228:i32)  [unwired: 1 out]
                n152 = property on="Test Ring" class="Ring (strict)"("Value"=w228, "Strings []"=w227) -> ()  [unwired: 2 in, 2 out]
                n153 = property on="Test Ring" class="Ring (strict)"("Visible"=TRUE) -> ()  [unwired: 2 in, 2 out]
                n154 = property on="Test Slider" class="Slide (strict)"("Visible"=FALSE) -> ()  [unwired: 2 in, 2 out]
              }
              frame "Exposure Priority  **" {
                n155 = Index Array(array=w239, index=3) -> (element=w240:cluster{string[]})
                n156 = call <vilib>:"NT Read String.vi"("name"=w242) -> ("value"=w241:string)  [unwired: 8 in, 2 out]
                n157 = Unbundle(w240) -> (w236:string[])
                n158 = Match First String(2:w236, 3:w241) -> (0:w237:i32)  [unwired: 1 out]
                n159 = property on="Test Ring" class="Ring (strict)"("Value"=w237, "Strings []"=w236) -> ()  [unwired: 2 in, 2 out]
                n160 = property on="Test Ring" class="Ring (strict)"("Visible"=TRUE) -> ()  [unwired: 2 in, 2 out]
                n161 = property on="Test Slider" class="Slide (strict)"("Visible"=FALSE) -> ()  [unwired: 2 in, 2 out]
              }
              frame "Color Enable  **" {
                n162 = Index Array(array=w248, index=4) -> (element=w249:cluster{string[]})
                n163 = call <vilib>:"NT Read String.vi"("name"=w251) -> ("value"=w250:string)  [unwired: 8 in, 2 out]
                n164 = Unbundle(w249) -> (w245:string[])
                n165 = Match First String(2:w245, 3:w250) -> (0:w246:i32)  [unwired: 1 out]
                n166 = property on="Test Ring" class="Ring (strict)"("Value"=w246, "Strings []"=w245) -> ()  [unwired: 2 in, 2 out]
                n167 = property on="Test Ring" class="Ring (strict)"("Visible"=TRUE) -> ()  [unwired: 2 in, 2 out]
                n168 = property on="Test Slider" class="Slide (strict)"("Visible"=FALSE) -> ()  [unwired: 2 in, 2 out]
              }
              frame Default {
                n169 = property on="Test Ring" class="Ring (strict)"("Visible"=FALSE) -> ()  [unwired: 2 in, 2 out]
                n170 = property on="Test Slider" class="Slide (strict)"("Visible"=FALSE) -> ()  [unwired: 2 in, 2 out]
              }
              frame "Brightness  **", "Color Level  **", "Compression  **", "FPS  **", "Sharpness  **" {
                n171 = call <vilib>:"NT Read Number.vi"("name"=w257) -> ("value"=w256:dbl)  [unwired: 8 in, 2 out]
                n172 = local write "Test Slider"(w256) -> ()
                n173 = property on="Test Slider" class="Slide (strict)"("Visible"=TRUE, "Scale.Maximum"=100.0 ("Scale.Range:Maximum")) -> ()  [unwired: 2 in, 2 out]
                n174 = property on="Test Ring" class="Ring (strict)"("Visible"=FALSE) -> ()  [unwired: 2 in, 2 out]
              }
            }
          }
        }
        n175 = property on="Progress" class="Clust (strict)"("Visible"=FALSE) -> ()  [unwired: 2 in, 2 out]
      }
      event "Test Name": Mouse Enter {
        # "Populate the ring with the list of tests"
        n176 = event-data() -> ()  [unwired: 1 in, 1 out]
        n177 = call <vilib>:"NT Read String Array.vi"("name"="TestMode/TestList" ("Name")) -> ("value"=w264:string[])  [unwired: 8 in, 2 out]
        n178 = Build Array (concatenate)("Select the test to run...", w264) -> (w263:string[])
        n179 = property on="Test Name" class="Ring (strict)"("Strings []"=w263) -> ()  [unwired: 2 in, 2 out]
      }
      event "Test Name": Value Change {
        w265 = FALSE ("Visible")
        # "Tell the robot the test name to run"
        n180 = event-data() -> ("NewVal"=w269:u16)  [unwired: 1 in]
        n181 = property on="Test Name" class="Ring (strict)"() -> ("Strings []"=w270:string[])  [unwired: 2 in, 2 out]
        n182 = local write "Progress"(T5 {"Test Progress"=0, "Test Progress Text"=""} ("Progress")) -> ()
        n183 = Index Array(array=w270, index=w269) -> (element=w268:string)
        n184 = call <vilib>:"NT Write String.vi"("value"=w268, "name"="TestMode/TestName" ("Name")) -> ()  [unwired: 9 in, 1 out]
        n185 = property on="Progress" class="Clust (strict)"("Visible"=TRUE) -> ()  [unwired: 2 in, 2 out]
        n186 = property on="Motor" class="Clust (strict)"("Visible"=w265) -> ()  [unwired: 2 in, 2 out]
        n187 = property on="Test Slider" class="Slide (strict)"("Visible"=w265) -> ()  [unwired: 2 in, 2 out]
        n188 = property on="On/Off" class="Bool (strict)"("Visible"=w265) -> ()  [unwired: 2 in, 2 out]
        n189 = property on="Rev/Fwd" class="Clust (strict)"("Visible"=w265) -> ()  [unwired: 2 in, 2 out]
        n190 = property on="Test Ring" class="Ring (strict)"("Visible"=w265) -> ()  [unwired: 2 in, 2 out]
      }
      event "Select Auto": Mouse Enter {
        # "Populate the combo box with the list of autonomous options"
        n191 = event-data() -> ()  [unwired: 1 in, 1 out]
        n192 = call <vilib>:"NT Read String Array.vi"("name"="Auto List" ("Name")) -> ("value"=w272:string[])  [unwired: 8 in, 2 out]
        n193 = property on="Select Auto" class="CmbBox"("Strings[]"=w272) -> ()  [unwired: 2 in, 2 out]
      }
      event "Select Auto": Value Change {
        # "User modified the Auto Selection. Write to NT variable so robot knows."
        n194 = event-data() -> ("NewVal"=w274:string)  [unwired: 1 in]
        n195 = call <vilib>:"NT Write String.vi"("value"=w274, "name"="Auto Selector" ("Name")) -> ()  [unwired: 9 in, 1 out]
      }
      event "CheckList": Double Click {
        # "Shift clears all"
        # "Update symbols on the listbox"
        n196 = event-data() -> ("PlatMods.Shift"=w276:bool, "Row"=w278:i32)  [unwired: 1 in]
        n197 = case shown="True" w276 {
          tunnel: w278 -> [w282 _]
          tunnel: 1 -> [w281 _]
          frame False {
            n198 = property on="CheckList" class="LstBox (strict)"() -> ("Item Symbols"=w280:i32[])  [unwired: 2 in, 2 out]
            n199 = Replace Array Subset(array=w280, new element=w281, index=w282) -> (w279:i32[])
            n200 = property on="CheckList" class="LstBox (strict)"("Item Symbols"=w279) -> ()  [unwired: 2 in, 2 out]
          }
          frame True {
            w283 = 0 ("Top Row")
            n201 = property on="CheckList" class="LstBox (strict)"() -> ("Number of Rows"=w285:u32)  [unwired: 2 in, 2 out]
            n202 = Initialize Array(0, w285) -> (w284:i32[])
            n203 = property on="CheckList" class="LstBox (strict)"("Top Row"=w283, "Value"=w283, "Item Symbols"=w284) -> ()  [unwired: 2 in, 2 out]
          }
        }
      }
      event "CheckList": Key Down {
        # "Update symbols on the listbox\nLeft and right keys check and uncheck"
        n204 = event-data() -> ("VKey"=w288:T21)  [unwired: 1 in]
        n205 = case shown="\"Left\", \"Right\"" w288 {
          selector: w288 -> [w293 _]
          tunnel: eventvkey."Left" ("VKey") -> [w291 _]
          frame "Left", "Right" {
            n206 = Equal?(x=w291, y=w293) -> (x = y?=w292:bool)
            n207 = Select(t=0, s=w292, f=1) -> (s? t:f=w294:i32)
            n208 = property on="CheckList" class="LstBox (strict)"() -> ("Item Symbols"=w297:i32[])  [unwired: 2 in, 2 out]
            n209 = Replace Array Subset(array=w297, new element=w294, index="CheckList") -> (w296:i32[])
            n210 = property on="CheckList" class="LstBox (strict)"("Item Symbols"=w296) -> ()  [unwired: 2 in, 2 out]
          }
          frame Default {
          }
        }
      }
      event "Motor.Enable": Value Change {
        # "When the test mode otor enable helper is set, update that\ntree row item's value"
        n211 = event-data() -> ("NewVal"=w302:bool)  [unwired: 1 in]
        n212 = Unbundle("Motor") -> ("Value"=w301:dbl)  [unwired: 1 out]
        n213 = Select(t=w301, s=w302, f=0.0) -> (s? t:f=w299:dbl)
        n214 = call <vilib>:"NT Write Number.vi"("value"=w299, "name"=w298) -> ()  [unwired: 9 in, 1 out]
      }
      event "Test Slider": Value Change {
        # "When the test mode slider helper is set, update that\ntree row item's value"
        n215 = event-data() -> ("NewVal"=w304:dbl)  [unwired: 1 in]
        n216 = call <vilib>:"NT Write Number.vi"("value"=w304, "name"=w305) -> ()  [unwired: 9 in, 1 out]
      }
      event "On/Off": Value Change {
        # "When the test mode on/off helper value is set, update that\ntree row item's value"
        n217 = event-data() -> ("NewVal"=w308:bool)  [unwired: 1 in]
        n218 = Boolean To (0,1)(Boolean=w308) -> (0, 1=w307:i16)
        n219 = call <vilib>:"NT Write Number.vi"("value"=w307, "name"=w306) -> ()  [unwired: 9 in, 1 out]
      }
      event "Rev/Fwd": Value Change {
        # "When the test mode helper value for relays is set, update that\ntree row item's value"
        n220 = event-data() -> ("NewVal.Forward"=w315:bool, "NewVal.Reverse"=w314:bool)  [unwired: 1 in]
        n221 = Boolean To (0,1)(Boolean=w315) -> (0, 1=w311:i16)
        n222 = Boolean To (0,1)(Boolean=w314) -> (0, 1=w313:i16)
        n223 = Negate(x=w313) -> (-x=w312:i16)
        n224 = Add(x=w311, y=w312) -> (x+y=w310:i16)
        n225 = call <vilib>:"NT Write Number.vi"("value"=w310, "name"=w309) -> ()  [unwired: 9 in, 1 out]
      }
      event "Test Ring": Value Change {
        # "When a test mode helper value is selected from the ring,\nset the tree item's variable to the string value"
        n226 = event-data() -> ("NewVal"=w318:u16)  [unwired: 1 in]
        n227 = property on="Test Ring" class="Ring (strict)"() -> ("Strings []"=w319:string[])  [unwired: 2 in, 2 out]
        n228 = Index Array(array=w319, index=w318) -> (element=w317:string)
        n229 = call <vilib>:"NT Write String.vi"("value"=w317, "name"=w316) -> ()  [unwired: 9 in, 1 out]
      }
      event "Rec Mode": Value Change {
        # "Update globals for recording mode and path to read log from.\nClear when logging and let NetworkTables set path for vision to\nuse."
        n230 = event-data() -> ("NewVal"=w328:enum32{"Stop", "Record", "Playback"})  [unwired: 1 in]
        n231 = global write "WPI_DashboardLogging Global.vi" "Logging Filename"(path "") -> ()
        n232 = global write "WPI_DashboardLogging Global.vi" "Recording"(w328) -> ()
        n233 = case shown="\"Playback\"" w328 {
          tunnel: w327 -> [_ w330 w338]
          tunnel: [_ _ w337] -> w325
          tunnel: [_ _ w336] -> _
          tunnel: w323 -> [_ _ w334]
          tunnel: cluster{i32, i32} {-250, 170} -> [_ _ w333]
          tunnel: [_ _ T22 {"Image Size"=TRUE, "Image Type"=TRUE, "Pixel Value"=TRUE, "ROI Information"=TRUE, "Zoom Factor"=FALSE} ("Image Information Shown:All Elements")] -> w320
          tunnel: [_ _ TRUE ("Zoom Factor")] -> w321
          frame Default {
          }
          frame "Stop", "Record" {
            # "Place Window too"
            n234 = invoke class="VI" method="FP.Close"(reference=w330) -> (reference out=w329:refnum<vi>)  [unwired: 2 in, 2 out]
            n235 = invoke class="VI" method="Abort VI"(reference=w329) -> ()  [unwired: 2 in, 3 out]
          }
          frame "Playback" {
            n236 = call "Open Playback Panel.vi"("Offset"=w333, "DB VI Ref"=w334, "Playback in"=w338) -> ("Playback out"=w335:refnum<vi>)  [unwired: 8 in]
            n237 = register-events(w335) -> (reference out=w337:refnum<event-registration>, error out=w336:errorcluster)  [unwired: 2 in]
          }
        }
        n238 = property on="Camera Image" class="ImageControl"("Image Information Shown"=w320, "Image Information Visible"=w321) -> ()  [unwired: 2 in, 2 out]
        n239 = call <vilib>:"WPI_DashboardNT Log FieldName Cache.vi"("Operation"=enum16{"Lookup/Add", "Index", "Clear"}."Clear") -> ()  [unwired: 8 in, 3 out]
      }
      event Panel Close {
        w339 = enum32{"Stop", "Record", "Playback"}."Stop" ("Rec Mode")
        # "Playback window has been closed, abort"
        n240 = event-data() -> ()  [unwired: 1 in, 4 out]
        n241 = local write "Rec Mode"(w339) -> ()
        n242 = global write "WPI_DashboardLogging Global.vi" "Recording"(w339) -> ()
      }
      event Panel Close {
        # "Abort playback window and ourself"
        n243 = event-data() -> ()  [unwired: 1 in, 4 out]
        n244 = invoke class="VI" method="FP.Close"(reference=w342) -> (reference out=w341:refnum<vi>)  [unwired: 2 in, 2 out]
        n245 = invoke class="VI" method="Abort VI"(reference=w341) -> (error out=w340:errorcluster)  [unwired: 2 in, 2 out]
        n246 = invoke class="VI" method="Abort VI"(error in=w340) -> ()  [unwired: 2 in, 3 out]
      }
      event "Tree": Double Click {
        n247 = event-data() -> ("PlatMods"=w348:T24, "Tag"=w345:string)  [unwired: 1 in]
        n248 = Unbundle(w348) -> ("Shift"=w347:bool)  [unwired: 4 out]
        n249 = String Subset(string=w345, length (rest)=1 ("length (rest)")) -> (substring=w344:string)  [unwired: 1 in]
        n250 = Not(x=w347) -> (.not. x?=w346:bool)
        n251 = case shown="\"/\"" w344 {
          tunnel: w345 -> [_ w350]
          tunnel: w346 -> [_ w349]
          frame Default {
          }
          frame "/" {
            n252 = call <vilib>:"NT Update Persistence.vi"("Persistence"=w349, "Name"=w350) -> ()  [unwired: 9 in, 1 out]
          }
        }
      }
    }
  }
  n253 = while {
    tunnel: w44 -> [w352]
    i -> [w355]
    stop <- FALSE stop-if-true
    n254 = Wait (ms)(milliseconds to wait=u32 100) -> ()  [unwired: 1 out]
    n255 = case shown="\"Playback\"" "Rec Mode" {
      tunnel: w355 -> [_ _ w370]
      tunnel: [u32 2829099 ("Base Color") u32 11141120 ("Target Color") w359] -> w351
      frame "Stop", Default {
        # "Reset the color, extra updates don't cost much"
      }
      frame "Record" {
      }
      frame "Playback" {
        # "Playback"
        n256 = Quotient & Remainder(x=w370, y=u32 50 ("milliseconds to wait")) -> (x-y*floor(x/y)=w366:u32)  [unwired: 1 out]
        n257 = Divide(x=w366, y=u32 50 ("milliseconds to wait")) -> (x/y=w363:dbl)
        n258 = Multiply(x=6.283185307179586, y=w363) -> (x*y=w368:dbl)
        n259 = Sine(x=w368) -> (sin(x)=w367:dbl)
        n260 = Absolute Value(x=w367) -> (abs(x)=w360:dbl)
        n261 = call "Interpolate RGB Color.vi"("Proportion"=w360, "Target Color"=u32 30976, "Base Color"=u32 2829099) -> ("Result Color"=w359:u32)  [unwired: 8 in]
      }
    }
    n262 = property class="Pane"(reference=w352, "PaneColor"=w351) -> ()  [unwired: 1 in, 2 out]
  }
  n263 = local write "Dashboard Tab"(T2."Drive" ("Dashboard Tab")) -> ()
  n264 = property on="On/Off" class="Bool (strict)"("Visible"=w17) -> ()  [unwired: 2 in, 2 out]
  n265 = property on="Motor" class="Clust (strict)"("Visible"=w17) -> ()  [unwired: 2 in, 2 out]
  n266 = property on="Progress" class="Clust (strict)"("Visible"=w17) -> ()  [unwired: 2 in, 2 out]
  n267 = property on="Test Ring" class="Ring (strict)"("Visible"=w17) -> ()  [unwired: 2 in, 2 out]
  n268 = property on="Rev/Fwd" class="Clust (strict)"("Visible"=w17) -> ()  [unwired: 2 in, 2 out]
  n269 = while {
    tunnel: u16 1741 ("timeout ms (25000)") -> [w372]
    stop <- FALSE stop-if-true
    n270 = TCP Create Listener(10:w372) -> (0:w371:errorcluster, 3:w373:refnum<k5>)  [unwired: 4 in, 1 out]
    n271 = case shown="No Error" w371 {
      selector: w371 -> [w375 _]
      tunnel: w373 -> [w376 _]
      frame No Error {
        n272 = while {
          tunnel: w376 -> [w379]
          tunnel: w375 -> [w378]
          stop <- FALSE stop-if-true
          n273 = TCP Wait On Listener(8:w378, 11:w379) -> (0:w380:errorcluster, 4:w381:refnum<k5>)  [unwired: 2 in, 3 out]
          n274 = local write "TCP"(w381) -> ()
          n275 = case shown="Error" w380 {
            frame No Error {
            }
            frame Error {
              n276 = Wait (ms)(milliseconds to wait=u32 1000) -> ()  [unwired: 1 out]
            }
          }
        }
      }
      frame Error {
        n277 = Wait (ms)(milliseconds to wait=u32 1000) -> ()  [unwired: 1 out]
      }
    }
  }
  n278 = global write "WPI_DashboardLogging Global.vi" "Recording"(w39) -> ()
  n279 = local write "Rec Mode"(w39) -> ()
  n280 = call <vilib>:"NT Write String.vi"("value"="Select Auto", "name"="Auto Selector" ("Name")) -> ()  [unwired: 9 in, 1 out]
